vi "zad7.vi"() -> ()   [LabVIEW 2017]
panel:
  out "XY Graph":cluster{"Y":dbl[], "Y":dbl[]}[](graph)
  out "Array":dbl[](array[numeric])
  in  "Numeric":dbl
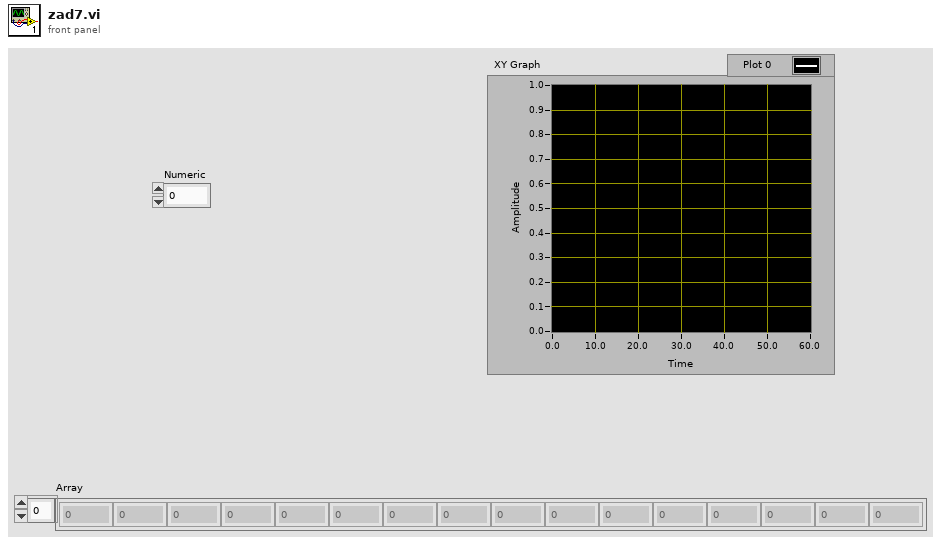
[diagram p1: front panel]
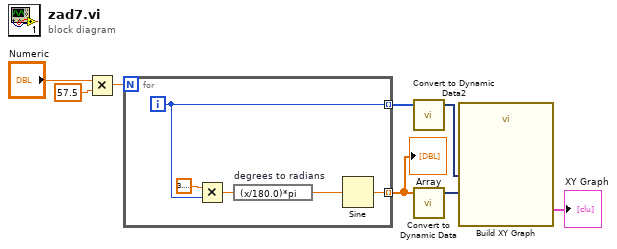
[diagram p0: block diagram]
diagram:
  n1 = Multiply(x="Numeric", y=57.5 ("Numeric 2")) -> (x*y=w2:dbl)
  n2 = for {
    N: w2 -> [_]
    tunnel: [w12] -> w1 mode=indexing
    tunnel: [w11] -> w6 mode=indexing
    i -> [w11]
    n3 = Multiply(x=3.141592653589793, y=w11) -> (x*y=w10:dbl)
    n4 = expression code="(x/180.0)*pi" "degrees to radians"(w10) -> (w9:dbl)
    n5 = Sine(x=w9) -> (sin(x)=w12:dbl)
  }
  "Array" <- w1
  n6 = call "Convert to Dynamic Data2"("Array"=w6) -> ("Dynamic Data Type"=w5:dynamicdata)  [unwired: 3 in]
  n7 = call "Convert to Dynamic Data"("Array"=w1) -> ("Dynamic Data Type"=w7:dynamicdata)  [unwired: 3 in]
  n8 = call "Build XY Graph"("Y Input"=w7, "X Input"=w5) -> ("XY Graph"=→"XY Graph":cluster{"X":dbl[], "Y":dbl[]}[])  [unwired: 8 in, 1 out]
